vi "tcs shm put Sample kernel Pointing Model LV.vi"(8 "error in (no error)":errorcluster, 11 "kernel_PointingModel_Ctl":T1) -> (0 "error out":errorcluster, 2 "function return":i32, 3 "kernel_PointingModel_Ctl out":T1)   [LabVIEW 2016, in "SALLV_tcs.lvlib"]
doc: "int tcs_shm_putSample_kernel_PointingModelLV(tcs_kernel_PointingModelLV *kernel_PointingModel_Ctl );"
uses:
  SALLV_tcs.lvlib
  SALLV_tcs.so
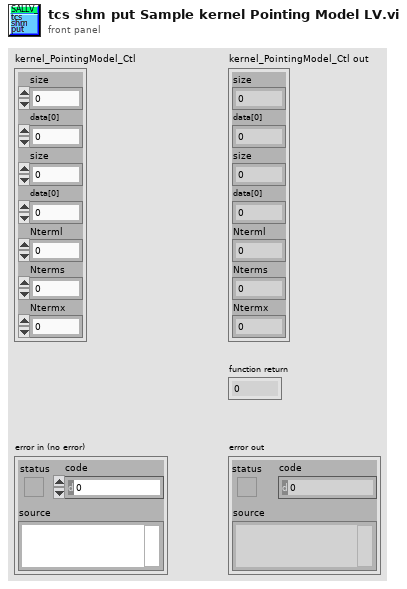
[diagram p1: front panel]
types:
  T1 = cluster{"size":i32, "data[0]":sgl, "size":i32, "data[0]":i32, "Nterml":i32, "Nterms":i32, "Ntermx":i32}
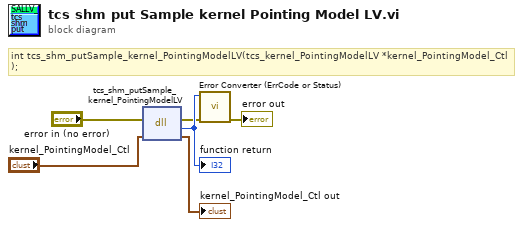
[diagram p0: block diagram]
diagram:
  # "int tcs_shm_putSample_kernel_PointingModelLV(tcs_kernel_PointingModelLV *kernel_PointingModel_Ctl );"
  n1 = dll-call lib="home/andres/Desktop/SALLV_tcs/SALLV_tcs.*" fn="tcs_shm_putSample_kernel_PointingModelLV"(error in="error in (no error)", "kernel_PointingModel_Ctl"="kernel_PointingModel_Ctl") -> (error out=w2:errorcluster, w6:i32, "kernel_PointingModel_Ctl"=→"kernel_PointingModel_Ctl out":T1)  [unwired: 2 in, 1 out]
  "function return" <- w6
  n2 = call "Error Converter (ErrCode or Status).vi"("error in (no error)"=w2, "error code"=w6) -> ("error out"=→"error out":errorcluster)  [unwired: 9 in]
